vi "ke37xx Self-Test.vi"(0 "VISA resource name":refnum<visa-resource-name>, 7 "Timeout (40 sec)":u32=40000, 11 "error in (no error)":errorcluster) -> (4 "VISA resource name out":refnum<visa-resource-name>, 8 "Self-Test Error":u32, 10 "Self-Test Response":string, 15 "error out":errorcluster)   [LabVIEW 2009, in "Keithley 3700 Series.lvlib"]
doc: "This VI causes the instrument to perform a self-test and returns the results. A numeric indicator indicates if the instrument passed all self-tests, and a string indicator contains the instrument's reponse."
uses:
  <instrlib>/Keithley 3706/Keithley 3700 Series.lvlib
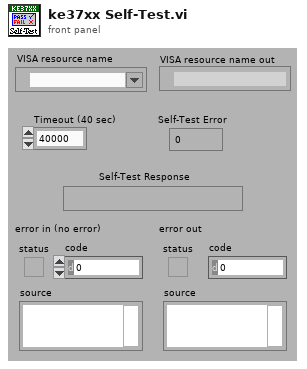
[diagram p1: front panel]
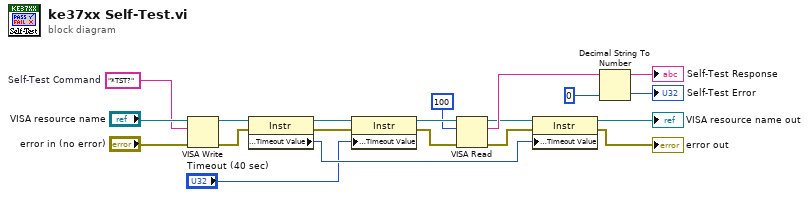
[diagram p0: block diagram]
diagram:
  w4 = "*TST?"  # Self-Test Command
  n1 = VISA Write(VISA resource name="VISA resource name", write buffer=w4, error in (no error)="error in (no error)") -> (VISA resource name out=w13:refnum<visa-resource-name>, error out=w14:errorcluster)  [unwired: 1 out]
  n2 = property class="Instr"(reference=w13, error in=w14) -> (reference out=w12:refnum<visa-resource-name>, error out=w11:errorcluster, "General Settings:Timeout Value"=w7:u32)
  n3 = property class="Instr"(reference=w12, error in=w11, "General Settings:Timeout Value"="Timeout (40 sec)") -> (reference out=w17:refnum<visa-resource-name>, error out=w16:errorcluster)
  n4 = VISA Read(VISA resource name=w17, byte count=u32 100 ("byte count (0)"), error in (no error)=w16) -> (VISA resource name out=w8:refnum<visa-resource-name>, read buffer=w10:string, error out=w9:errorcluster)  [unwired: 1 out]
  "Self-Test Response" <- w10
  n5 = property class="Instr"(reference=w8, error in=w9, "General Settings:Timeout Value"=w7) -> (reference out=→"VISA resource name out":refnum<visa-resource-name>, error out=→"error out":errorcluster)
  n6 = Decimal String To Number(string=w10, default (0L)=u32 0 ("Default (0L)")) -> (number=→"Self-Test Error":u32)  [unwired: 2 out]
